vi "get operating mode.vi"(8 "error in (no error)":errorcluster, 11 "LineCCD in":refnum<class "LineCCD.lvclass">) -> (0 "error out":errorcluster, 3 "LineCCD out":refnum<class "LineCCD.lvclass">)   [LabVIEW 2012, in "LineCCD.lvclass"]
uses:
  LineCCD.lvclass
  LineCCD.lvclass/LineCCD.ctl
  <instrlib>/ALPHALAS CCD S Series/ALPHALAS CCD S Series.lvlib
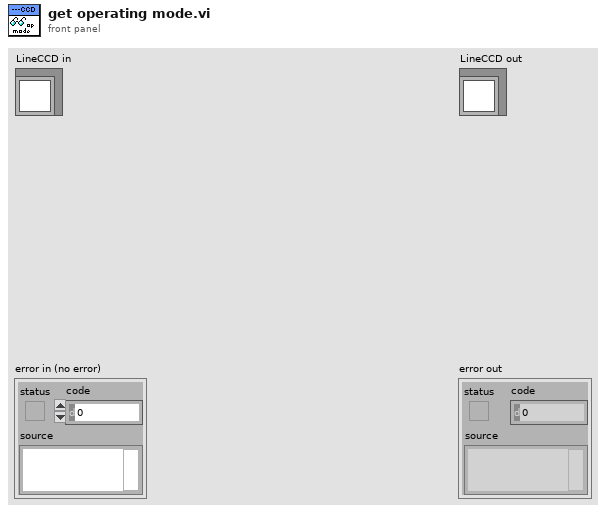
[diagram p1: front panel]
types:
  T1 = typedef "ALPHALAS CCD S Series.lvlib/Operating Mode.ctl" = u16
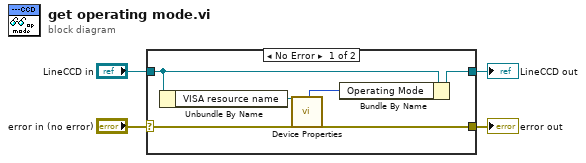
[diagram p0: block diagram]
diagram:
  n1 = case shown="No Error" "error in (no error)" {
    selector: "error in (no error)" -> [w7 w12]
    tunnel: [w6 w12] -> w3
    tunnel: [w8 w11] -> w1
    tunnel: "LineCCD in" -> [w9 w11]
    frame No Error {
      n2 = Unbundle By Name(w9) -> ("VISA resource name"=w10:refnum<visa-resource-name>)
      n3 = call <instrlib>:"Device Properties.vi"("VISA resource name"=w10, "error in (no error)"=w7) -> ("Operating Mode"=w5:T1, "error out"=w6:errorcluster)  [unwired: 6 in, 18 out]
      n4 = Bundle By Name(cluster=w9, "Operating Mode"=w5) -> (w8:refnum<class "LineCCD.lvclass">)
    }
    frame Error {
    }
  }
  "error out" <- w3
  "LineCCD out" <- w1
